vi "user-event.vi"() -> ()   [LabVIEW 2013]
panel:
  out "monitor event":refnum<user-event>
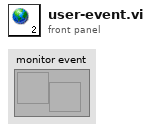
[diagram p1: front panel]
diagram:
